vi "instrument.Cryostation.Client.vi"(8 "error in (no error)":errorcluster, 9 "Data":variant, 10 "Command":T1, 11 "instrument.Cryostation in":refnum<class "instrument.Cryostation.lvclass">) -> (0 "error out":errorcluster, 1 "Data out":variant, 2 "Command out":string, 3 "instrument.Cryostation out":refnum<class "instrument.Cryostation.lvclass">)   [LabVIEW 2016, in "instrument.Cryostation.lvclass"]
uses:
  instrument.Cryostation.lvclass
  C:/Program Files (x86)/National Instruments/LabVIEW 2016/user.lib/LevyLab/Levylab Instruments/SMOs/Instrument/Instrument.lvclass
  Typedefs/Commands-enum.ctl
  <userlib>/LevyLab/Levylab Instruments/SMOs/Instrument/Instrument.lvclass
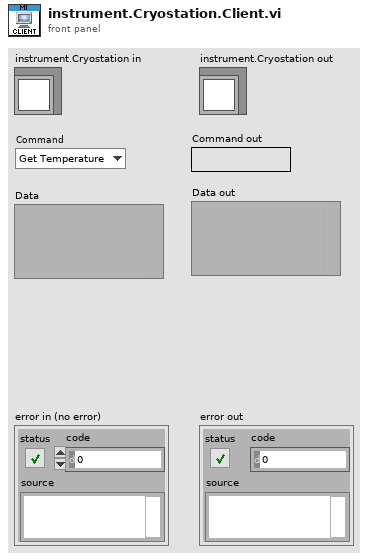
[diagram p1: front panel]
types:
  T1 = typedef "instrument.Cryostation.lvclass/Commands-enum.ctl" = enum16{"Get Temperature", "getAll"}
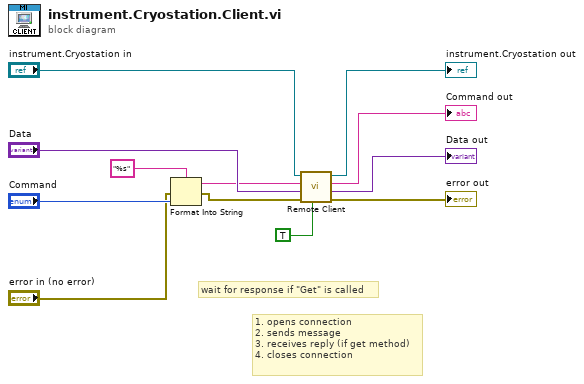
[diagram p0: block diagram]
diagram:
  # "1. opens connection\n2. sends message\n3. receives reply (if get method)\n4. closes connection"
  # "wait for response if \"Get\" is called"
  n1 = Format Into String(format string="%s", error in="error in (no error)", "Command") -> (resulting string=w4:string, error out=w1:errorcluster)  [unwired: 1 in]
  n2 = call <userlib>:"Remote Client.vi"("Wait for Response? [T]"=TRUE ("Wait for Response?"), "error in (no error)"=w1, "Data"="Data", "Command"=w4, "Instrument in"="instrument.Cryostation in") -> ("error out"=→"error out":errorcluster, "Data out"=→"Data out":variant, "Command out"=→"Command out":string, "Instrument out"=→"instrument.Cryostation out":refnum<class "instrument.Cryostation.lvclass">)  [unwired: 3 in]
